vi "get_status.vi"(7 "values":dbl[](array[numeric]), 8 "status in (low: False, high: True, medium: not changed)":bool[](array[boolean]), 9 "rules":T1(array[cluster])) -> (1 "msg to email":string, 2 "status out (low: False, high: True, medium: not changed)":bool[](array[boolean]), 3 "Alarms? array":bool[](array[boolean]))   [LabVIEW 2017]
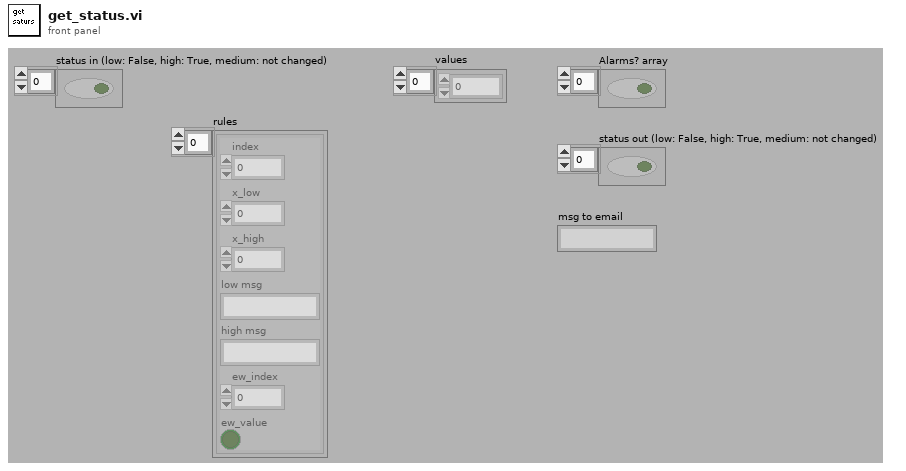
[diagram p1: front panel]
types:
  T1 = cluster{"index":i32, "x_low":dbl, "x_high":dbl, "low msg":string, "high msg":string, "ew_index":i32, "ew_value":bool}[]
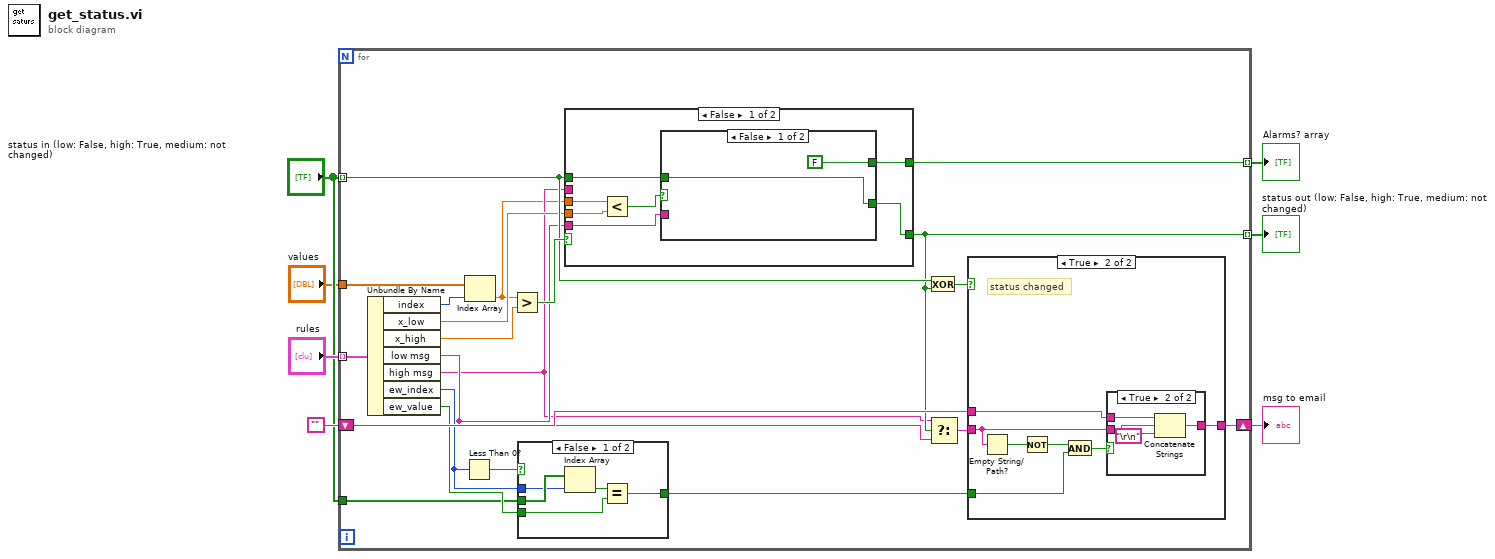
[diagram p0: block diagram]
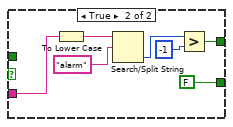
[diagram p3: hidden frame]
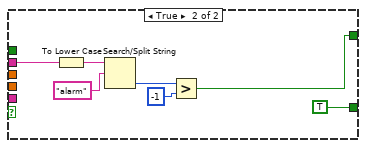
[diagram p4: hidden frame]
diagram:
  n1 = for {
    tunnel: "status in (low: False, high: True, medium: not changed)" -> [w23] mode=indexing
    shift-right: [w27] -> w5
    shift-left: "" -> [w26]
    tunnel: [w22] -> w6 mode=indexing
    tunnel: "rules" -> [w21] mode=indexing
    tunnel: [w20] -> w7 mode=indexing
    tunnel: "status in (low: False, high: True, medium: not changed)" -> [w13]
    tunnel: "values" -> [w10]
    n2 = Unbundle By Name(w21) -> ("index"=w9:i32, "x_low"=w19:dbl, "x_high"=w18:dbl, "low msg"=w17:string, "high msg"=w16:string, "ew_index"=w12:i32, "ew_value"=w14:bool)
    n3 = Less Than 0?(x=w12) -> (x < 0?=w15:bool)
    n4 = Index Array(array=w10, index=w9) -> (element=w8:dbl)
    n5 = Greater?(x=w8, y=w18) -> (0:w24:bool)
    n6 = case shown="False" w15 {
      selector: w15 -> [_ w34]
      tunnel: w14 -> [w30 _]
      tunnel: w13 -> [w33 _]
      tunnel: w12 -> [w32 _]
      tunnel: [w29 w34] -> w11
      frame False {
        n7 = Index Array(array=w33, index=w32) -> (element=w31:bool)
        n8 = Equal?(x=w31, y=w30) -> (x = y?=w29:bool)
      }
      frame True {
      }
    }
    n9 = case shown="False" w24 {
      tunnel: [w38 TRUE] -> w22
      tunnel: w8 -> [w41 _]
      tunnel: w23 -> [w39 _]
      tunnel: w19 -> [w37 _]
      tunnel: w17 -> [w36 _]
      tunnel: w16 -> [_ w52]
      tunnel: [w35 w51] -> w20
      frame False {
        n10 = Less?(x=w41, y=w37) -> (x < y?=w40:bool)
        n11 = case shown="False" w40 {
          tunnel: w36 -> [_ w45]
          tunnel: w39 -> [w43 _]
          tunnel: [w43 FALSE] -> w38
          tunnel: [FALSE w44] -> w35
          frame False {
          }
          frame True {
            n12 = To Lower Case(string=w45) -> (all lower case string=w49:string)
            n13 = Search/Split String(string=w49, search string/char (-)="alarm" ("搜索字符串/字符(-)")) -> (offset of match=w48:i32)  [unwired: 3 out]
            n14 = Greater?(x=w48, y=-1) -> (0:w44:bool)
          }
        }
      }
      frame True {
        n15 = To Lower Case(string=w52) -> (all lower case string=w55:string)
        n16 = Search/Split String(string=w55, search string/char (-)="alarm" ("搜索字符串/字符(-)")) -> (offset of match=w54:i32)  [unwired: 3 out]
        n17 = Greater?(x=w54, y=-1) -> (0:w51:bool)
      }
    }
    n18 = Exclusive Or(1:w22, 2:w23) -> (0:w28:bool)
    n19 = Select(t=w16, s=w22, f=w17) -> (s? t:f=w25:string)
    n20 = case shown="True" w28 {
      tunnel: w25 -> [_ w63]
      tunnel: [w58 w65] -> w27
      tunnel: w26 -> [w58 w64]
      tunnel: w11 -> [_ w60]
      frame False {
        # "status unchanged"
      }
      frame True {
        # "status changed"
        n21 = Empty String/Path?(string/path=w63) -> (empty?=w62:bool)
        n22 = Not(x=w62) -> (.not. x?=w61:bool)
        n23 = And(x=w61, y=w60) -> (x .and. y?=w59:bool)
        n24 = case shown="True" w59 {
          tunnel: [w66 w70] -> w65
          tunnel: w64 -> [w66 w69]
          tunnel: w63 -> [_ w68]
          frame False {
          }
          frame True {
            n25 = Concatenate Strings(w69, w68, "\r\n") -> (w70:string)
          }
        }
      }
    }
  }
  "Alarms? array" <- w7
  "status out (low: False, high: True, medium: not changed)" <- w6
  "msg to email" <- w5
